vi "TestForceGraph.vi"() -> ()   [LabVIEW 2017]
panel:
  out "Counter":dbl
  out "PeakForce":bool
  out "AngleMemory":dbl
  out "ForceMemory":dbl
  in  "Expand":bool
  out "ScanX 2":dbl
  out "ScanX":dbl
  in  "Auto":bool
  in  "First Touch":bool
  in  "Path":path
  in  "Filenames":string[](array[string])
  in  "FileType":string(combo)="DL"
  out "LED":bool
  out "Graph":cluster{"Y":dbl[], "Y":dbl[]}[](graph)
  # "RL\nUp/Down"
  # "RR\nUp/Down"
  # "FL\nUp/Down"
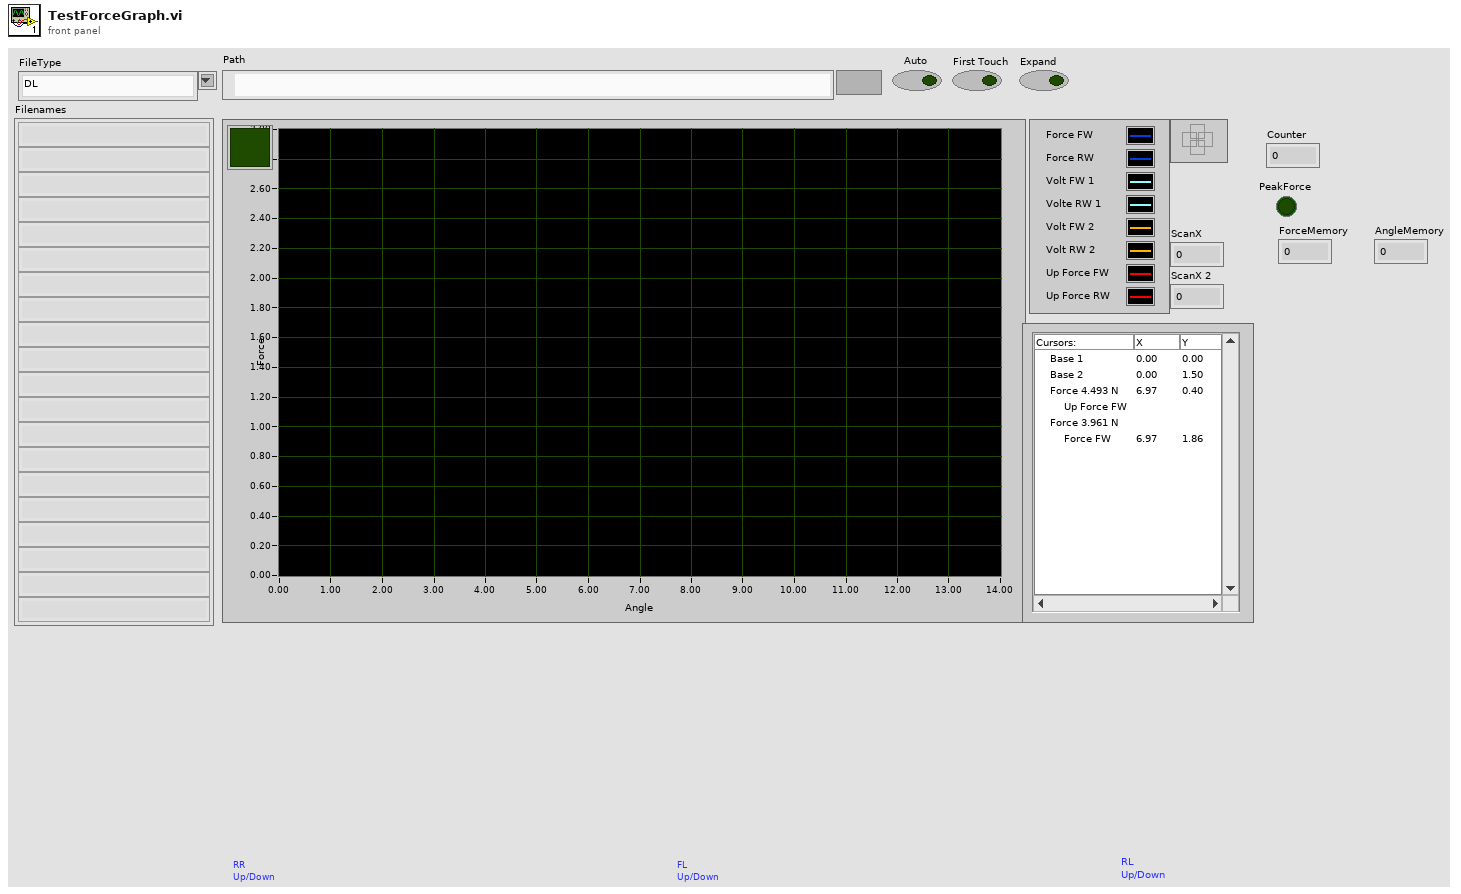
[diagram p1: front panel]
types:
  T1 = cluster{"DownMax":u16, "DownMin":u16, "UpMax":u16, "UpMin":u16}
  T2 = cluster{"Angle Data":dbl[], "Force Data":dbl[], "Volt Data 1":dbl[], "Volt Data 2":dbl[]}
  T3 = cluster{"Angle Data":dbl[], "Force Data 1":dbl[], "Force Data 2":dbl[], "Volt Data 1":dbl[], "Volt Data 2":dbl[]}
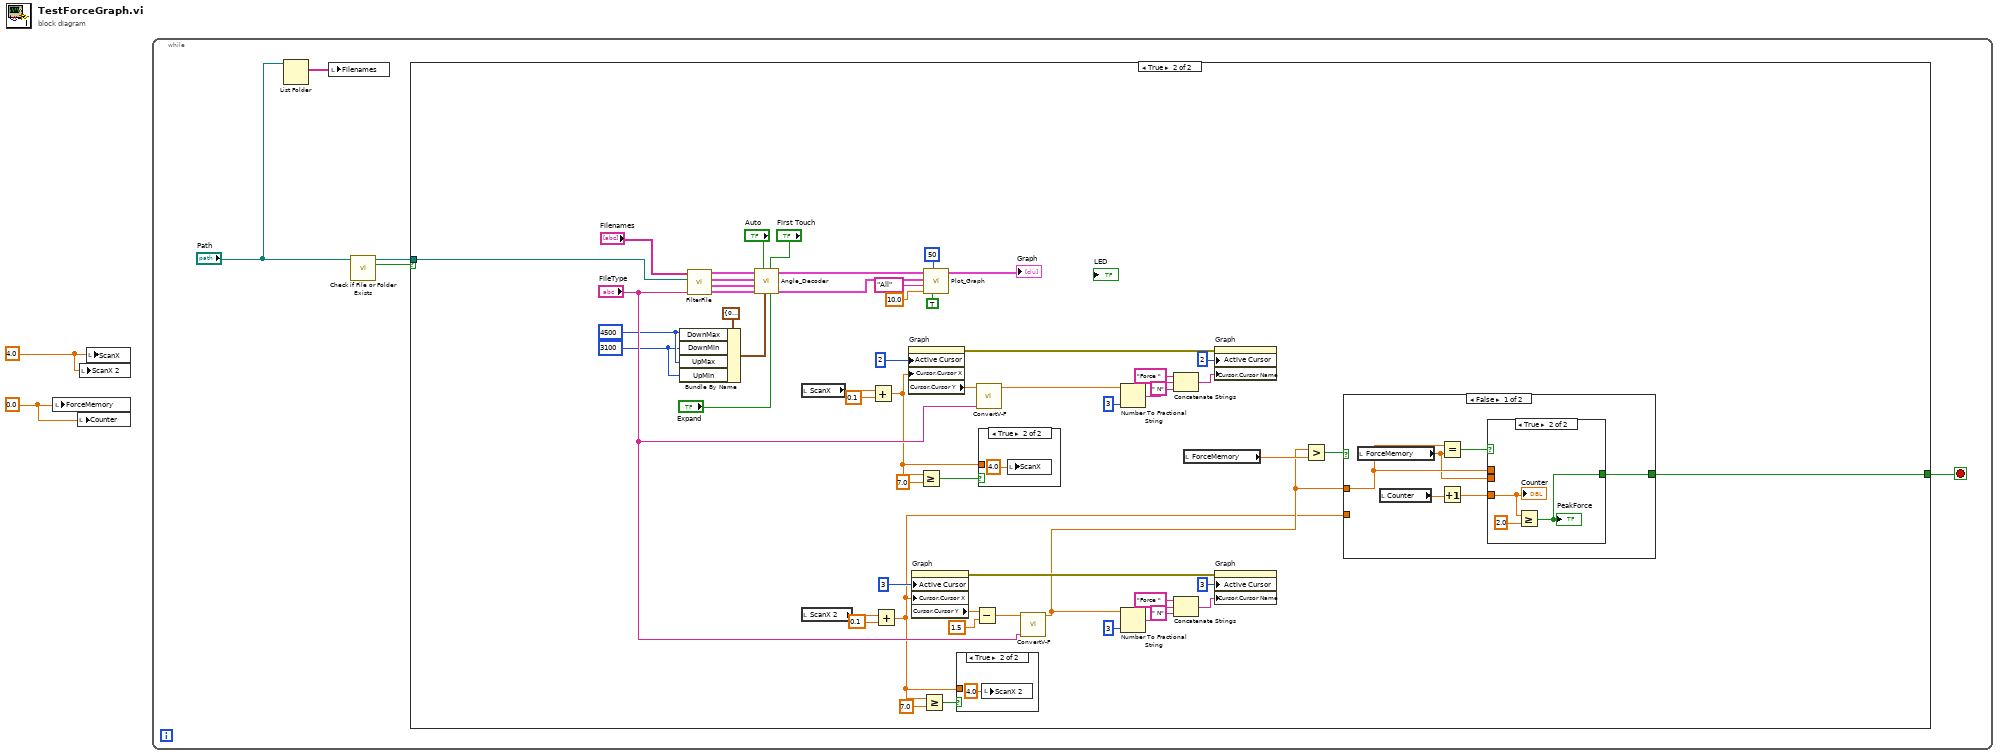
[diagram p0: block diagram]
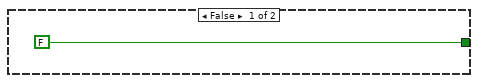
[diagram p2: hidden frame]
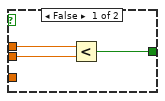
[diagram p3: hidden frame]
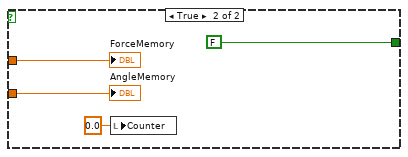
[diagram p4: hidden frame]
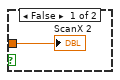
[diagram p5: hidden frame]
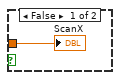
[diagram p6: hidden frame]
diagram:
  w1 = 0.0 ("ForceMemory")
  w2 = 4.0 ("ScanX 2")
  n1 = local write "ForceMemory"(w1) -> ()
  n2 = local write "Counter"(w1) -> ()
  n3 = local write "ScanX 2"(w2) -> ()
  n4 = local write "ScanX"(w2) -> ()
  n5 = while {
    stop <- w3 stop-if-true
    n6 = List Folder(path="Path") -> (filenames=w7:string[])  [unwired: 3 in, 3 out]
    n7 = local write "Filenames"(w7) -> ()
    n8 = call <vilib>:"Check if File or Folder Exists.vi"("path"="Path") -> ("file or folder exists?"=w6:bool, "dup path"=w4:path)  [unwired: 8 in, 1 out]
    n9 = case shown="True" w6 {
      tunnel: w4 -> [_ w53]
      tunnel: [FALSE w21] -> w3
      frame False {
      }
      frame True {
        w30 = u16 3100
        w31 = u16 4500
        n10 = Bundle By Name(cluster=T1 {"DownMax"=0, "DownMin"=0, "UpMax"=0, "UpMin"=0} ("AngleUpDown"), "DownMax"=w31, "DownMin"=w30, "UpMax"=w31, "UpMin"=w30) -> (w56:T1)
        n11 = call "FilterFile.vi"("FileType"="FileType", "Path"=w53, "Filenames"="Filenames") -> ("RW_Up"=w64:T2, "FW_Up"=w35:T2, "RW_Down"=w63:T2, "FW_Down"=w36:T2)  [unwired: 3 in, 2 out]
        n12 = call "Angle_Decoder.vi"("Expand"="Expand", "Find Fist Touch"="First Touch", "AngleUpDown"=w56, "Auto/Manual"="Auto", "Analog RW Up"=w64, "Analog FW Up"=w35, "Analog RW Down"=w63, "Analog FW Down"=w36) -> ("Analog RW D/U"=w33:T3, "Analog FW D/U"=w34:T3)  [unwired: 2 in]
        n13 = local read "ScanX"() -> (w49:dbl)
        n14 = local read "ScanX 2"() -> (w44:dbl)
        n15 = Add(x=w49, y=0.1) -> (x+y=w25:dbl)
        n16 = Add(x=w44, y=0.1) -> (x+y=w22:dbl)
        n17 = property on="Graph" class="XYGraph (strict)"("Active Cursor"=u32 2, "Cursor.Cursor X"=w25) -> (error out=w47:errorcluster, "Cursor.Cursor Y"=w24:dbl)  [unwired: 2 in, 1 out]
        n18 = property on="Graph" class="XYGraph (strict)"("Active Cursor"=u32 3, "Cursor.Cursor X"=w22) -> (error out=w40:errorcluster, "Cursor.Cursor Y"=w39:dbl)  [unwired: 2 in, 1 out]
        n19 = Greater Or Equal?(x=w25, y=7.0) -> (x >= y?=w50:bool)
        n20 = Greater Or Equal?(x=w22, y=7.0) -> (x >= y?=w43:bool)
        n21 = call "Plot_Graph.vi"("EnableSmooth"=TRUE, "FillZeroFirstSignal"=50, "VoltDevider"=10.0, "Channel"="All", "Analog RW In"=w33, "Analog FW In"=w34) -> ("XY Graph"=→"Graph":cluster{"Angle Data":dbl[], "Array":dbl[]}[])  [unwired: 5 in]
        n22 = case shown="True" w43 {
          tunnel: w22 -> [w81 _]
          frame False {
            "ScanX 2" <- w81
          }
          frame True {
            n23 = local write "ScanX 2"(4.0 ("ScanX")) -> ()
          }
        }
        n24 = Subtract(x=w39, y=1.5) -> (x-y=w37:dbl)
        n25 = call "ConvertV-F.vi"("Test Name"="FileType", "Volt In"=w24) -> ("Force Out"=w26:dbl)  [unwired: 9 in]
        n26 = case shown="True" w50 {
          tunnel: w25 -> [w83 _]
          frame False {
            "ScanX" <- w83
          }
          frame True {
            n27 = local write "ScanX"(4.0 ("ScanX")) -> ()
          }
        }
        n28 = call "ConvertV-F.vi"("Test Name"="FileType", "Volt In"=w37) -> ("Force Out"=w23:dbl)  [unwired: 9 in]
        n29 = Number To Fractional String(number=w26, precision (6)=i16 3) -> (F-format string=w13:string)  [unwired: 2 in]
        n30 = Number To Fractional String(number=w23, precision (6)=i16 3) -> (F-format string=w17:string)  [unwired: 2 in]
        n31 = Concatenate Strings("Force " ("string"), w13, " N" ("string")) -> (w10:string)
        n32 = Concatenate Strings("Force " ("string"), w17, " N" ("string")) -> (w20:string)
        n33 = local read "ForceMemory"() -> (w28:dbl)
        n34 = property on="Graph" class="XYGraph (strict)"(error in=w47, "Active Cursor"=u32 2, "Cursor.Cursor Name"=w10) -> ()  [unwired: 1 in, 2 out]
        n35 = property on="Graph" class="XYGraph (strict)"(error in=w40, "Active Cursor"=u32 3, "Cursor.Cursor Name"=w20) -> ()  [unwired: 1 in, 2 out]
        n36 = Greater?(x=w23, y=w28) -> (0:w27:bool)
        n37 = case shown="False" w27 {
          tunnel: w23 -> [w66 w80]
          tunnel: w22 -> [_ w79]
          tunnel: [w67 FALSE] -> w21
          frame False {
            n38 = local read "ForceMemory"() -> (w65:dbl)
            n39 = local read "Counter"() -> (w68:dbl)
            n40 = Equal?(x=w66, y=w65) -> (x = y?=w70:bool)
            n41 = Increment(x=w68) -> (x+1=w69:dbl)
            n42 = case shown="True" w70 {
              tunnel: w69 -> [_ w76]
              tunnel: [w73 w74] -> w67
              tunnel: w66 -> [w72 _]
              tunnel: w65 -> [w71 _]
              frame False {
                n43 = Less?(x=w72, y=w71) -> (x < y?=w73:bool)
              }
              frame True {
                n44 = Greater Or Equal?(x=w76, y=2.0) -> (x >= y?=w74:bool)
                "PeakForce" <- w74
                "Counter" <- w76
              }
            }
          }
          frame True {
            n45 = local write "Counter"(0.0 ("Counter")) -> ()
            "ForceMemory" <- w80
            "AngleMemory" <- w79
          }
        }
      }
    }
  }
